vi "CheckWIFIName.vi"(5 "Slot":T1, 7 "error out":errorcluster, 9 "WIFI":string) -> (0 "错误输出":errorcluster, 2 "比对结果":bool)   [LabVIEW 2013]
uses:
  SystemCode/SysControl/Slot.ctl
panel:
  out "提示":string
  out "Wi-FI名称":string
  in  "PASS":bool
  in  "停止":bool
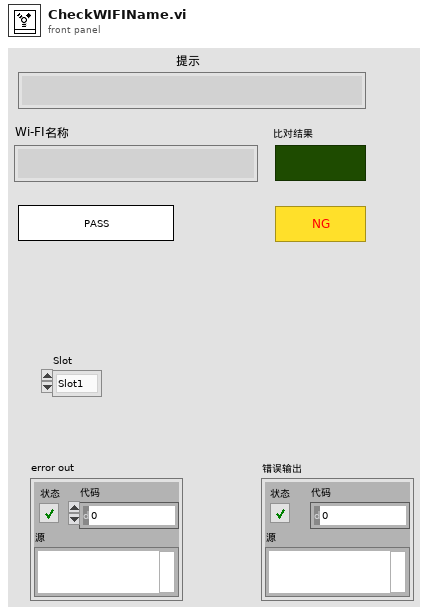
[diagram p1: front panel]
types:
  T1 = typedef "Slot.ctl" = enum16{"Slot1", "Slot2", "Slot3", "Slot4"}
  T2 = typedef "LVRectTypeDef.ctl" = cluster{"Left":i16, "Top":i16, "Right":i16, "Bottom":i16}
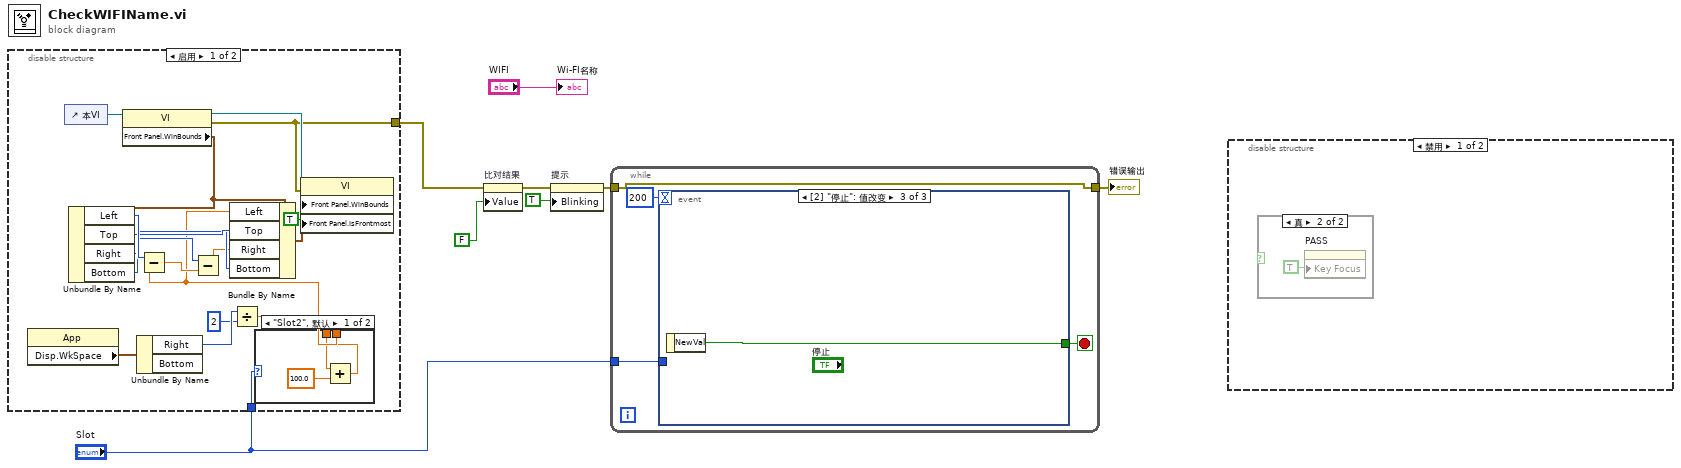
[diagram p0: block diagram]
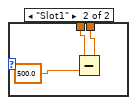
[diagram p4: hidden frame]
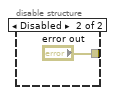
[diagram p5: hidden frame]
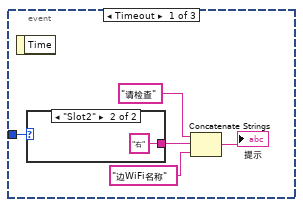
[diagram p6: hidden frame]
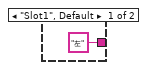
[diagram p7: hidden frame]
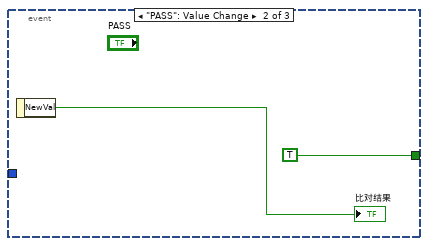
[diagram p8: hidden frame]
diagram:
  n1 = disable-structure shown="启用" {
    disable-tunnel: [w14 "error out"] -> w3
    disable-tunnel: "Slot" -> [w9 _]
    frame Enabled {
      n2 = property class="App"() -> ("Disp.WkSpace"=w23:T2)  [unwired: 2 in, 2 out]
      n3 = control-ref of="本VI"() -> (w26:refnum<vi>)
      n4 = property class="VI"(reference=w26) -> (reference out=w25:refnum<vi>, error out=w14:errorcluster, "Front Panel.WinBounds"=w21:T2)  [unwired: 1 in]
      n5 = Unbundle By Name(w21) -> ("Left"=w20:i16, "Top"=w19:i16, "Right"=w17:i16, "Bottom"=w18:i16)
      n6 = Unbundle By Name(w23) -> ("Right"=w13:i16)  [unwired: 1 out]
      n7 = Divide(x=w13, y=i16 2) -> (x/y=w11:dbl)
      n8 = case shown="\"Slot2\", 默认" w9 {
        tunnel: w11 -> [w29 w32]
        tunnel: [w27 w30] -> w10
        frame "Slot2", Default {
          n9 = Add(x=w29, y=100.0) -> (x+y=w27:dbl)
        }
        frame "Slot1" {
          n10 = Subtract(x=w32, y=500.0) -> (x-y=w30:dbl)
        }
      }
      n11 = Subtract(x=w20, y=w10) -> (x-y=w16:dbl)
      n12 = Subtract(x=w17, y=w16) -> (x-y=w15:dbl)
      n13 = Bundle By Name(cluster=w21, "Left"=w10, "Top"=w19, "Right"=w15, "Bottom"=w18) -> (w24:T2)
      n14 = property class="VI"(reference=w25, error in=w14, "Front Panel.WinBounds"=w24, "Front Panel.IsFrontmost"=TRUE ("前面板窗口:可调整大小")) -> ()  [unwired: 2 out]
    }
    frame Disabled {
    }
  }
  n15 = property on="比对结果" class="Bool (严格)"(error in=w3, "Value"=FALSE ("比对结果")) -> (error out=w5:errorcluster)  [unwired: 1 in, 1 out]
  n16 = property on="提示" class="Str"(error in=w5, "Blinking"=TRUE ("闪烁")) -> (error out=w8:errorcluster)  [unwired: 1 in, 1 out]
  n17 = while {
    tunnel: w8 -> [w35]
    tunnel: [w35] -> w4
    tunnel: "Slot" -> [w34]
    stop <- w37 stop-if-true
    n18 = event shown="[2] \"停止\": 值改变" {
      selector: _ -> [_ _ _]
      dyn-events: _ -> [_ _ _]
      timeout: 200 -> [_ _ _]
      tunnel: [_ TRUE w47] -> w37
      tunnel: w34 -> [w38 _ _]
      event Timeout {
        n19 = event-data() -> ()  [unwired: 1 in, 1 out]
        n20 = case shown="\"Slot2\"" w38 {
          tunnel: ["左" ("字符串") "右" ("字符串")] -> w39
          frame "Slot1", Default {
          }
          frame "Slot2" {
          }
        }
        n21 = Concatenate Strings("请检查" ("字符串"), w39, "边WiFi名称" ("字符串")) -> (→"提示":string)
      }
      event "PASS": Value Change {
        n22 = event-data() -> ("NewVal"=→"比对结果":bool)  [unwired: 1 in]
      }
      event "停止": Value Change {
        n23 = event-data() -> ("NewVal"=w47:bool)  [unwired: 1 in]
      }
    }
  }
  "错误输出" <- w4
  n24 = disable-structure shown="禁用" {
    frame Disabled {
      n25 = case shown="真" {
        selector: _ -> [_ _]
        frame False {
        }
        frame True {
          n26 = property on="PASS" class="Bool"("Key Focus"=TRUE ("键选中")) -> ()  [unwired: 2 in, 2 out]
        }
      }
    }
    frame Enabled {
    }
  }
  "Wi-FI名称" <- "WIFI"
